vi "Fit Data.vi"(8 "error in":errorcluster, 10 "Data In":dbl[](array[numeric]), 11 "DFT-5 in":refnum<class "DFT5.lvclass">) -> (0 "error out":errorcluster, 3 "DFT-5 out":refnum<class "DFT5.lvclass">)   [LabVIEW 2016, in "Exponential Fit Library.lvlib" / "DFT5.lvclass"]
doc: "Calculate tau from a weighting of the first five components of the DFT using the weights given in the initialization structure. The frequency components are calculated as described in DFT-1 and then averaged according to the equation\n\nbeta_mean = sum(beta_k*weight_k)/sum(weight_k)\n\nThe scale (A) and offset (B) are calculated as:\n\nA = (w^2+k^2)/ k*Re[F(n=1)]*dt/(1-exp(-k*tm)\nB = F(0)/N - A/(k*tm)*[1-exp(-k*tm)]\n\nwhere N is the number of samples, k = 1/tau, w = omega = 2*pi/tm, tm = N*dt, F(0) is the DC component of the FFT and Re[F(n=1)] is the real term of the first frequency component in the FFT spectrum. These computations are taken from Mazurenka et al. (2005) and are used in the determination of the uncertainty in the term tau (e_tau)."
uses:
  DFT5.lvclass
  G:/sw_repo/For Builds/Reusable/General/Math/Fit Exponential Class/Fit Exponential.lvclass
  Fit Exponential.lvclass/Fit Exponential.ctl
  DFT5.lvclass/DFT5.ctl
  <vilib>/Analysis/2dsp.llb/Real FFT.vi
  Read Size.vi
  Read Sin.vi
  Read Cos.vi
  Read Weights.vi
  Read Weight Sum.vi
  Get Dt.vi
  Write Output.vi
  Fit Exponential.lvclass
  <vilib>/Analysis/NI_AALPro.lvlib
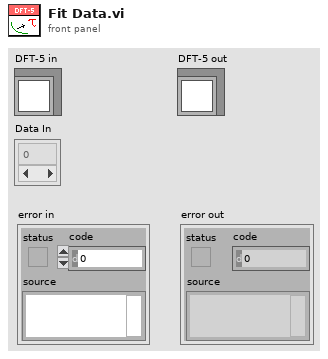
[diagram p1: front panel]
types:
  T1 = cluster{"A":dbl, "B":dbl, "tau":dbl, "e_tau":dbl}
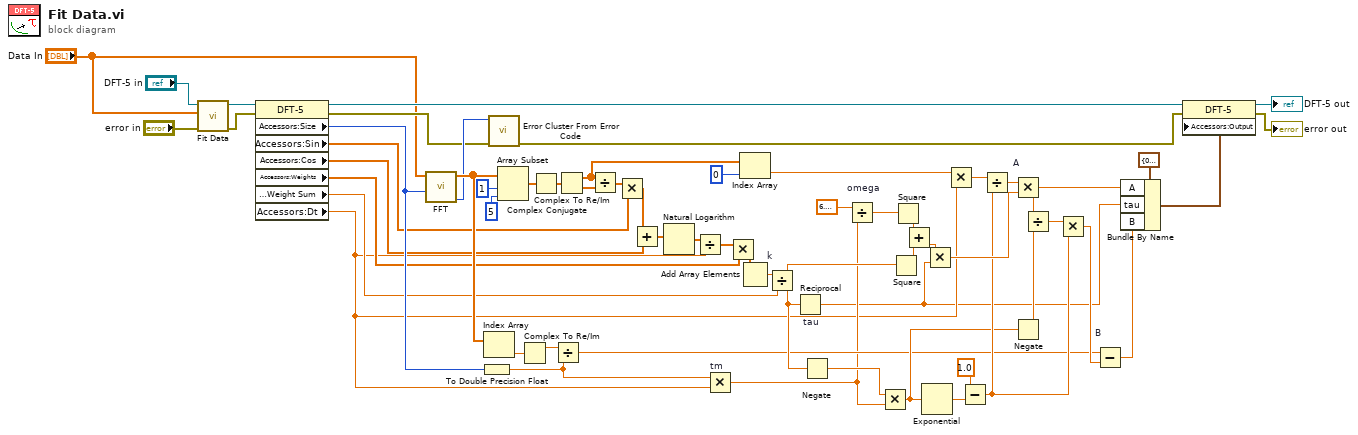
[diagram p0: block diagram]
diagram:
  n1 = call-parent "Fit Data.vi"("error in"="error in", "Data In"="Data In", "Fit Exponential in"="DFT-5 in") -> ("error out"=w1:errorcluster, "Fit Exponential out"=w2:refnum<class "DFT5.lvclass">)  [unwired: 7 in]
  n2 = property class="DFT-5"(reference=w2, error in=w1) -> (reference out=w14:refnum<class "DFT5.lvclass">, error out=w16:errorcluster, "Accessors:Size"=w21:i32, "Accessors:Sin"=w20:dbl[], "Accessors:Cos"=w19:dbl[], "Accessors:Weights"=w18:dbl[], "Accessors:Weight Sum"=w17:dbl, "Accessors:Dt"=w15:dbl)
  n3 = call-poly <vilib>:"FFT.vi"("FFT size"=w21, "X"="Data In") -> ("error"=w23:i32, "FFT {X}"=w33:cdb[])  [unwired: 1 in, 7 out]
  n4 = To Double Precision Float(number=w21) -> (double precision float=w22:dbl)
  n5 = Index Array(array=w33) -> (element=w32:cdb)  [unwired: 1 in]
  n6 = call <vilib>:"Error Cluster From Error Code.vi"("error in (no error)"=w16, "error code (0)"=w23) -> ("error out"=w12:errorcluster)  [unwired: 7 in]
  n7 = Array Subset(array=w33, index=1, length=5) -> (w55:cdb[])
  n8 = Complex To Re/Im(x + iy=w32) -> (x=w31:dbl)  [unwired: 1 out]
  n9 = Complex Conjugate(1:w55) -> (0:w53:cdb[])
  n10 = Divide(x=w31, y=w22) -> (x/y=w30:dbl)
  n11 = Complex To Re/Im(x + iy=w53) -> (x=w26:dbl[], y=w54:dbl[])
  n12 = Divide(x=w26, y=w54) -> (x/y=w46:dbl[])
  n13 = Multiply(x=w46, y=w20) -> (x*y=w58:dbl[])
  n14 = Add(x=w58, y=w19) -> (x+y=w57:dbl[])
  n15 = Natural Logarithm(1:w57) -> (0:w56:dbl[])
  n16 = Divide(x=w56, y=w15) -> (x/y=w50:dbl[])
  n17 = Multiply "tm"(x=w22, y=w15) -> (x*y=w29:dbl)
  n18 = Multiply(x=w50, y=w18) -> (x*y=w52:dbl[])
  n19 = Index Array(array=w26, index=0) -> (element=w25:dbl)
  n20 = Add Array Elements(numeric array=w52) -> (sum=w51:dbl)
  n21 = Divide "k"(x=w51, y=w17) -> (x/y=w45:dbl)
  n22 = Reciprocal "tau"(x=w45) -> (1/x=w8:dbl)
  n23 = Negate(x=w45) -> (-x=w44:dbl)
  n24 = Divide "omega"(x=6.283185307179586, y=w29) -> (x/y=w27:dbl)
  n25 = Multiply(x=w44, y=w29) -> (x*y=w37:dbl)
  n26 = Square(x=w45) -> (x^2=w49:dbl)
  n27 = Square(x=w27) -> (x^2=w48:dbl)
  n28 = Add(x=w48, y=w49) -> (x+y=w47:dbl)
  n29 = Exponential(1:w37) -> (0:w43:dbl)
  n30 = Multiply(x=w47, y=w8) -> (x*y=w40:dbl)
  n31 = Multiply(x=w25, y=w15) -> (x*y=w41:dbl)
  n32 = Subtract(x=1.0, y=w43) -> (x-y=w38:dbl)
  n33 = Divide(x=w41, y=w38) -> (x/y=w39:dbl)
  n34 = Multiply "A"(x=w39, y=w40) -> (x*y=w9:dbl)
  n35 = Negate(x=w37) -> (-x=w36:dbl)
  n36 = Divide(x=w9, y=w36) -> (x/y=w35:dbl)
  n37 = Multiply(x=w35, y=w38) -> (x*y=w34:dbl)
  n38 = Subtract "B"(x=w30, y=w34) -> (x-y=w7:dbl)
  n39 = Bundle By Name(cluster=T1 {"A"=0.0, "B"=0.0, "tau"=0.0, "e_tau"=0.0} ("Output"), "A"=w9, "tau"=w8, "B"=w7) -> (w6:T1)
  n40 = property class="DFT-5"(reference=w14, error in=w12, "Accessors:Output"=w6) -> (reference out=→"DFT-5 out":refnum<class "DFT5.lvclass">, error out=→"error out":errorcluster)
